vi "Format Data Buffer to Cluster.vi"(9 "tag_data_out":dbl[](array[numeric])) -> (1 "Analog Sensors":T1 {"Fuel Temp" scale=0.0..150.0 scale format="%#.1f"; "Flow(lbs/hr)" scale=0.0..1000.0 scale format="%#.1f"; "BP Monitor" scale=0.0..10.0 scale format="%#.1f"; "Bypass Pressure (psig)" scale=0.0..50.0 scale format="%#.1f"; "(Not Used)" scale=0.0..200.0 scale format="%#.1f"; "Back Pressure" scale=0.0..300.0 scale format="%#.1f"; "Diff. Pressure  (60 psid)" scale=0.0..60.0 scale format="%#.1f"; "Supply Pressure" scale=0.0..400.0 scale format="%#.1f"}, 3 "Actual Current":dbl)   [LabVIEW 2018]
uses:
  Controls/Gauge TDef.ctl
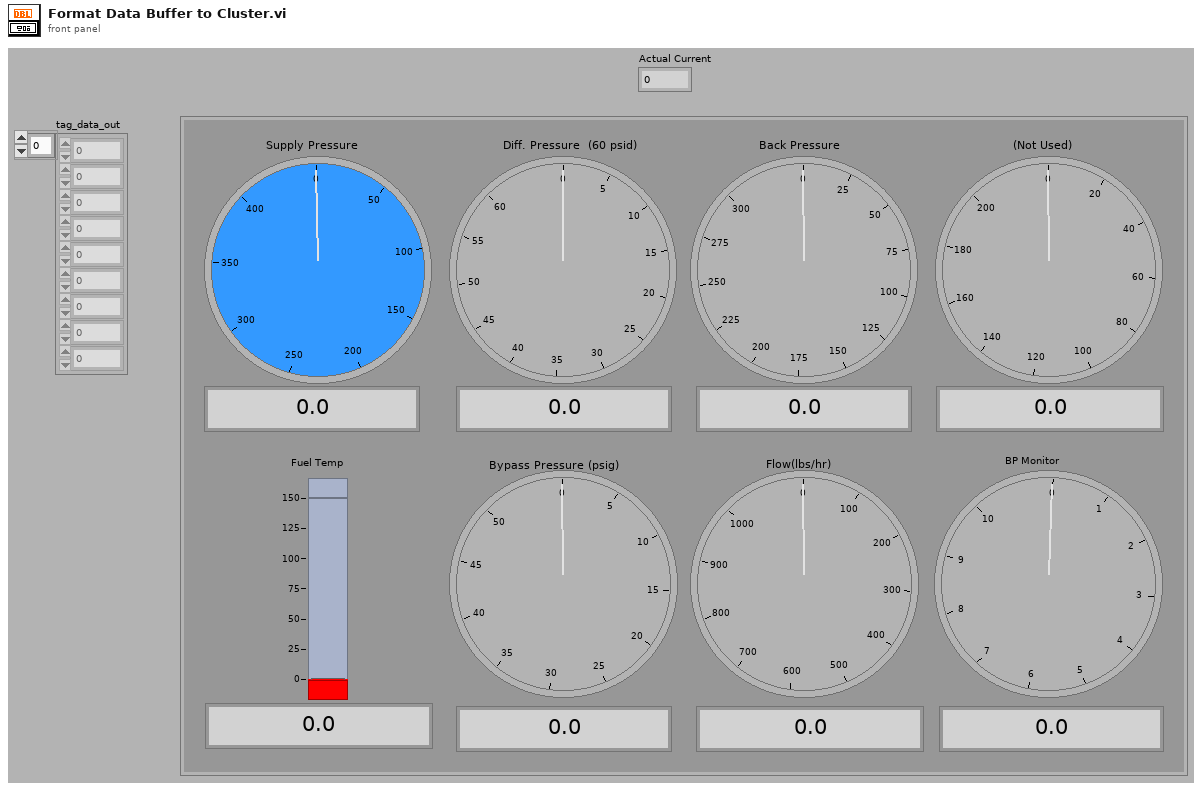
[diagram p1: front panel]
types:
  T1 = typedef "Gauge TDef.ctl" = cluster{"Flow(lbs/hr)":dbl, "Fuel Temp":dbl, "Supply Pressure":dbl, "Diff. Pressure  (60 psid)":dbl, "Back Pressure":dbl, "(Not Used)":dbl, "Bypass Pressure (psig)":dbl, "BP Monitor":dbl}
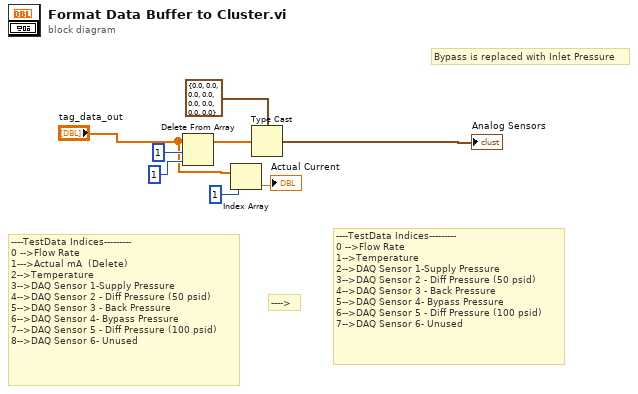
[diagram p0: block diagram]
diagram:
  # "Bypass is replaced with Inlet Pressure"
  # "---->"
  # "----TestData Indices---------\n0 -->Flow Rate\n1-->Temperature\n2-->DAQ Sensor 1-Supply Pressure\n3-->DAQ Sensor 2 - Diff Pressure (50 psid)\n4-->DAQ Sensor 3 - Back Pressure\n5-->DAQ Sensor 4- Bypass Pressure\n6-->DAQ Sensor 5 - Diff Pressure (100 psid)\n7-->DAQ Sensor 6- Unused"
  # "----TestData Indices---------\n0 -->Flow Rate\n1--->Actual mA  (Delete)\n2-->Temperature\n3-->DAQ Sensor 1-Supply Pressure\n4-->DAQ Sensor 2 - Diff Pressure (50 psid)\n5-->DAQ Sensor 3 - Back Pressure\n6-->DAQ Sensor 4- Bypass Pressure\n7-->DAQ Sensor 5 - Diff Pressure (100 psid)\n8-->DAQ Sensor 6- Unused"
  n1 = Delete From Array(array="tag_data_out", length=1, index=1) -> (array with subset deleted=w3:dbl[])  [unwired: 1 out]
  n2 = Index Array(array="tag_data_out", index=1) -> (element=→"Actual Current":dbl)
  n3 = Type Cast(type=T1 {"Flow(lbs/hr)"=0.0, "Fuel Temp"=0.0, "Supply Pressure"=0.0, "Diff. Pressure  (60 psid)"=0.0, "Back Pressure"=0.0, "(Not Used)"=0.0, "Bypass Pressure (psig)"=0.0, "BP Monitor"=0.0} ("Analog Sensors"), x=w3) -> (*(type *) &x=→"Analog Sensors":T1)
